vi "GetExperimentClass.vi"(8 "error in (no error)":errorcluster caption="entrée d'erreur (pas d'erreur)", 11 "Interface en entrée":refnum<class "Interface.lvclass">) -> (0 "error out":errorcluster caption="sortie d'erreur", 2 "Experiment.lvclass":refnum<class "Experiment.lvclass">, 3 "Interface en sortie":refnum<class "Interface.lvclass">)   [LabVIEW 2019, in "Interface.lvclass"]
uses:
  Interface.lvclass
  Experiment Class/Experiment.lvclass
  Interface.lvclass/Interface.ctl
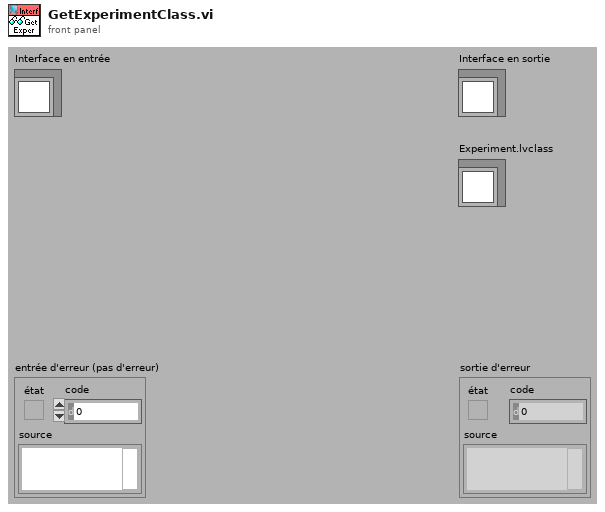
[diagram p1: front panel]
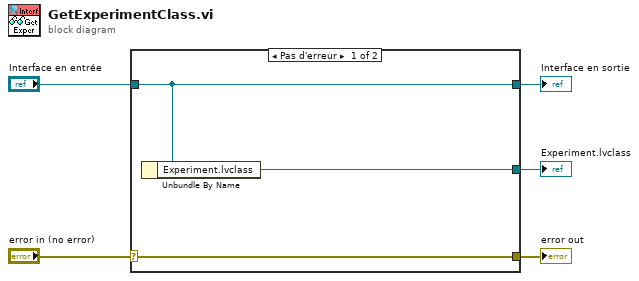
[diagram p0: block diagram]
diagram:
  n1 = case shown="Pas d'erreur" "error in (no error)" {
    selector: "error in (no error)" -> [w8 w9]
    tunnel: [w8 w9] -> w4
    tunnel: [w7 w10] -> w2
    tunnel: "Interface en entrée" -> [w7 w10]
    tunnel: [w6 _] -> w1
    frame No Error {
      n2 = Unbundle By Name(w7) -> ("Experiment.lvclass"=w6:refnum<class "Experiment.lvclass">)
    }
    frame Error {
    }
  }
  "error out" <- w4
  "Interface en sortie" <- w2
  "Experiment.lvclass" <- w1
